vi "WWorWD.vi"(11 "strModelChoice":string(combo)="WD5500") -> (1 "strOutput":string, 3 "WWorWD":bool)   [LabVIEW 2011]
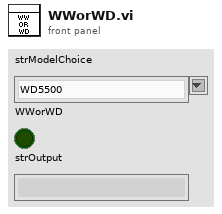
[diagram p1: front panel]
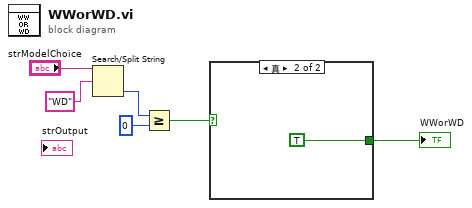
[diagram p0: block diagram]
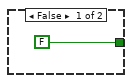
[diagram p2: hidden frame]
diagram:
  n1 = Search/Split String(string="strModelChoice", search string/char (-)="WD" ("搜索字符串/字符(-)")) -> (offset of match=w2:i32)  [unwired: 1 in, 2 out]
  n2 = Greater Or Equal?(x=w2, y=0) -> (x >= y?=w4:bool)
  n3 = case shown="真" w4 {
    tunnel: [FALSE TRUE] -> w5
    frame False {
    }
    frame True {
    }
  }
  "WWorWD" <- w5
